vi "Configure Channel Probe.vi"(4 "Probe Model Number (0: P5205)":i32(ring) items=["P5205", "P5210", "P6205", "P6241", "P6243", "P6245", "P6246", "P6247", "P6248", "P6249", "P6250", "P6251", "P670X", "P671X", "TCP202"], 5 "Set Probe Model Number (F: Disable)":bool, 6 "Probe Signal Type (1: Single-ended)":i32(ring)=1 items=["Differential", "Single-ended"], 7 "Skew Factor (1E-7 S)":dbl=1e-07, 8 "error in (no error)":errorcluster, 9 "Probe Head Type (8: NONE)":i32(ring)=8 items=["Single- ended, 0dB", "Single- ended, 6dB", "Single- ended, 12dB", "Single- ended, 20dB", "Differential, 0dB", "Differential, 6dB", "Differential, 12dB", "Differential, 20dB", "NONE", "Differential SMA probe head, 0 dB", "Differential SMA probe head, 6 dB"], 10 "Channel Name (0: Channel 1)":i32(ring) items=["Channel 1", "Channel 2", "Channel 3", "Channel 4"], 11 "VISA resource name":refnum<visa-resource-name>) -> (0 "error out":errorcluster, 3 "VISA resource name out":refnum<visa-resource-name>)   [LabVIEW 2017, in "Agilent 2000 3000 X-Series.lvlib"]
doc: "Configures the channel probe."
uses:
  Agilent 2000 3000 X-Series.lvlib
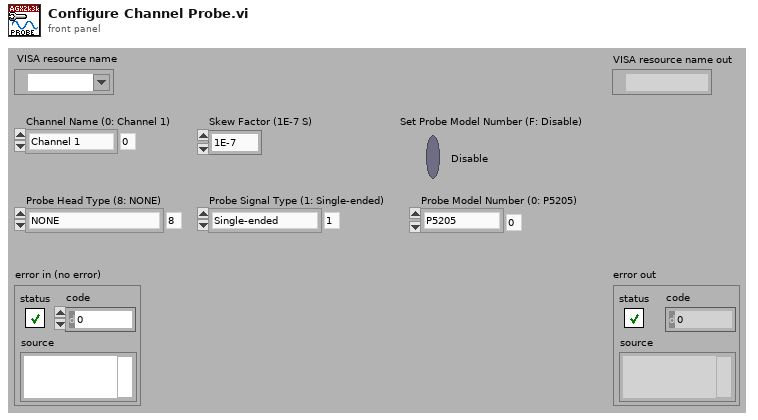
[diagram p1: front panel]
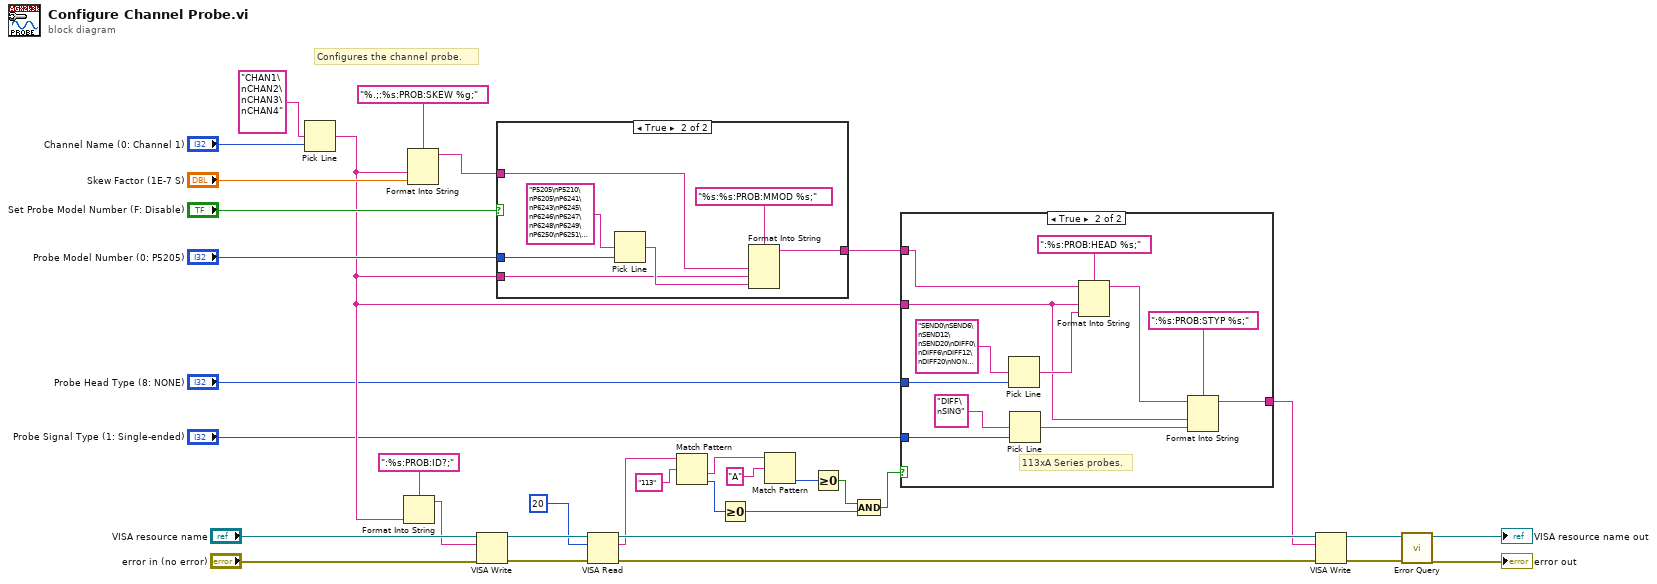
[diagram p0: block diagram]
diagram:
  # "Configures the channel probe."
  n1 = Pick Line(multi-line string="CHAN1\nCHAN2\nCHAN3\nCHAN4", line index="Channel Name (0: Channel 1)") -> (output string=w6:string)  [unwired: 1 out]
  n2 = Format Into String(format string=":%s:PROB:ID?;", w6) -> (resulting string=w20:string)  [unwired: 2 in, 1 out]
  n3 = Format Into String(format string="%.;:%s:PROB:SKEW %g;", w6, "Skew Factor (1E-7 S)") -> (resulting string=w24:string)  [unwired: 2 in, 1 out]
  n4 = VISA Write(VISA resource name="VISA resource name", write buffer=w20, error in (no error)="error in (no error)") -> (VISA resource name out=w19:refnum<visa-resource-name>, error out=w18:errorcluster)  [unwired: 1 out]
  n5 = case shown="True" "Set Probe Model Number (F: Disable)" {
    tunnel: [w35 w39] -> w3
    tunnel: "Probe Model Number (0: P5205)" -> [_ w42]
    tunnel: w6 -> [_ w38]
    tunnel: w24 -> [w35 w36]
    frame False {
    }
    frame True {
      n6 = Pick Line(multi-line string="P5205\nP5210\nP6205\nP6241\nP6243\nP6245\nP6246\nP6247\nP6248\nP6249\nP6250\nP6251\nP670X\nP671X\nTCP202", line index=w42) -> (output string=w40:string)  [unwired: 1 in]
      n7 = Format Into String(format string="%s:%s:PROB:MMOD %s;", w36, w38, w40) -> (resulting string=w39:string)  [unwired: 2 in, 1 out]
    }
  }
  n8 = VISA Read(VISA resource name=w19, byte count=u32 20, error in (no error)=w18) -> (VISA resource name out=w16:refnum<visa-resource-name>, read buffer=w14:string, error out=w15:errorcluster)  [unwired: 1 out]
  n9 = Match Pattern(string=w14, regular expression="113") -> (after substring=w11:string, offset past match=w1:i32)  [unwired: 1 in, 2 out]
  n10 = Greater Or Equal To 0?(x=w1) -> (x >= 0?=w9:bool)
  n11 = Match Pattern(string=w11, regular expression="A") -> (offset past match=w10:i32)  [unwired: 1 in, 3 out]
  n12 = Greater Or Equal To 0?(x=w10) -> (x >= 0?=w8:bool)
  n13 = Compound Arithmetic op=AND(w8, w9) -> (w7:bool)
  n14 = case shown="True" w7 {
    tunnel: w6 -> [_ w44]
    tunnel: "Probe Head Type (8: NONE)" -> [_ w52]
    tunnel: "Probe Signal Type (1: Single-ended)" -> [_ w51]
    tunnel: [w43 w46] -> w2
    tunnel: w3 -> [w43 w45]
    frame False {
    }
    frame True {
      # "113xA Series probes."
      n15 = Pick Line(multi-line string="SEND0\nSEND6\nSEND12\nSEND20\nDIFF0\nDIFF6\nDIFF12\nDIFF20\nNONE\nDSMA\nDSMA6", line index=w52) -> (output string=w55:string)  [unwired: 1 out]
      n16 = Pick Line(multi-line string="DIFF\nSING", line index=w51) -> (output string=w48:string)  [unwired: 1 out]
      n17 = Format Into String(format string=":%s:PROB:HEAD %s;", initial string=w45, w44, w55) -> (resulting string=w49:string)  [unwired: 1 in, 1 out]
      n18 = Format Into String(format string=":%s:PROB:STYP %s;", initial string=w49, w44, w48) -> (resulting string=w46:string)  [unwired: 1 in, 1 out]
    }
  }
  n19 = VISA Write(VISA resource name=w16, write buffer=w2, error in (no error)=w15) -> (VISA resource name out=w32:refnum<visa-resource-name>, error out=w31:errorcluster)  [unwired: 1 out]
  n20 = call "Error Query.vi"("error in (no error)"=w31, "VISA resource name"=w32) -> ("error out"=→"error out":errorcluster, "VISA resource name out"=→"VISA resource name out":refnum<visa-resource-name>)  [unwired: 8 out]
